vi "Material-Line1-Aquisition.vi"(8 "error in (no error)":errorcluster, 11 "Material-RunTest in":refnum<class "Material-RunTest.lvclass">) -> (0 "error out":errorcluster, 3 "Material-RunTest out":refnum<class "Material-RunTest.lvclass">)   [LabVIEW 2014, in "Material-RunTest.lvclass"]
uses:
  Material-RunTest.lvclass
  Material-RunTest.lvclass/Material-RunTest.ctl
  <instrlib>/Keyence LK-G5000/Public/enum/LKIF_OUTNO.ctl
  <vilib>/Utility/file.llb/Write To Spreadsheet File (DBL).vi
  <instrlib>/Keyence LK-G5000/Keyence LK-G5000.lvlib
  Motion Control/Motion-ControlAll.lvclass
  <vilib>/addons/_LabVIEW Style Book/Utilities/Style Book Utilities.lvlib
panel:
  out "Laser Value":sgl format="%_6g"
  out "Init Meas1":dbl[](array[numeric])
  out "stop collecting":bool=TRUE
  out "Meas 1 Dyn Data":dbl[](graph)
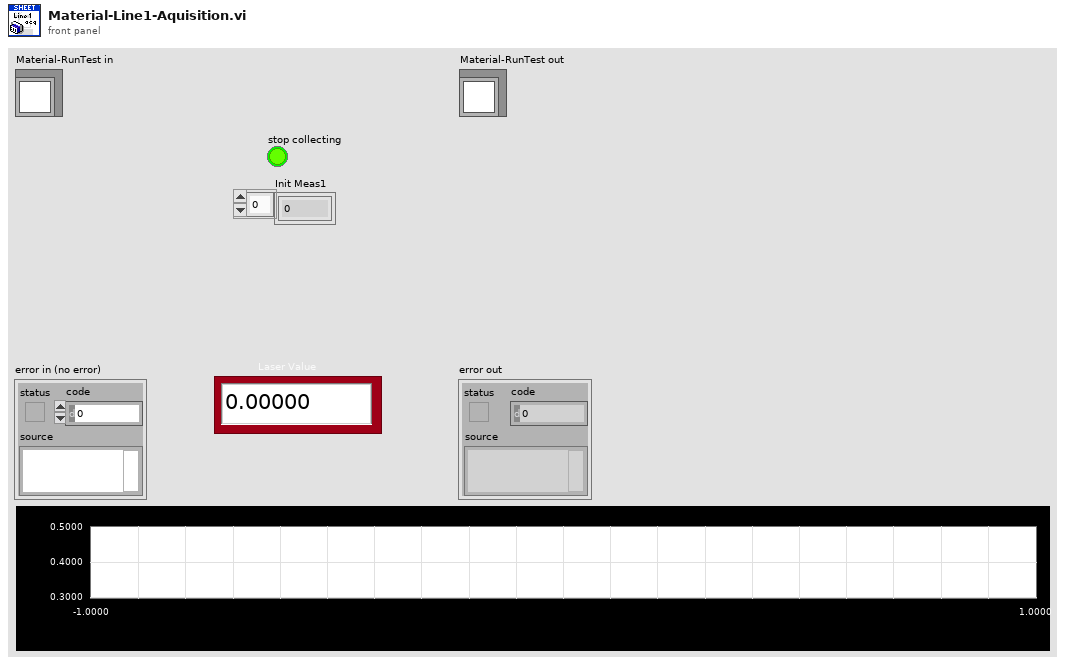
[diagram p1: front panel]
types:
  T1 = typedef "Keyence LK-G5000.lvlib/LKIF_OUTNO.ctl" = i32
  T2 = typedef "Keyence LK-G5000.lvlib/LKIF_FLOATRESULT.ctl" = i32
  T3 = cluster{"OutNo":i32, "LKIF_FLOATRESULT":T2, "Value":sgl}[]
  T4 = cluster{"OutNo":i32, "LKIF_FLOATRESULT":T2, "Value":sgl}
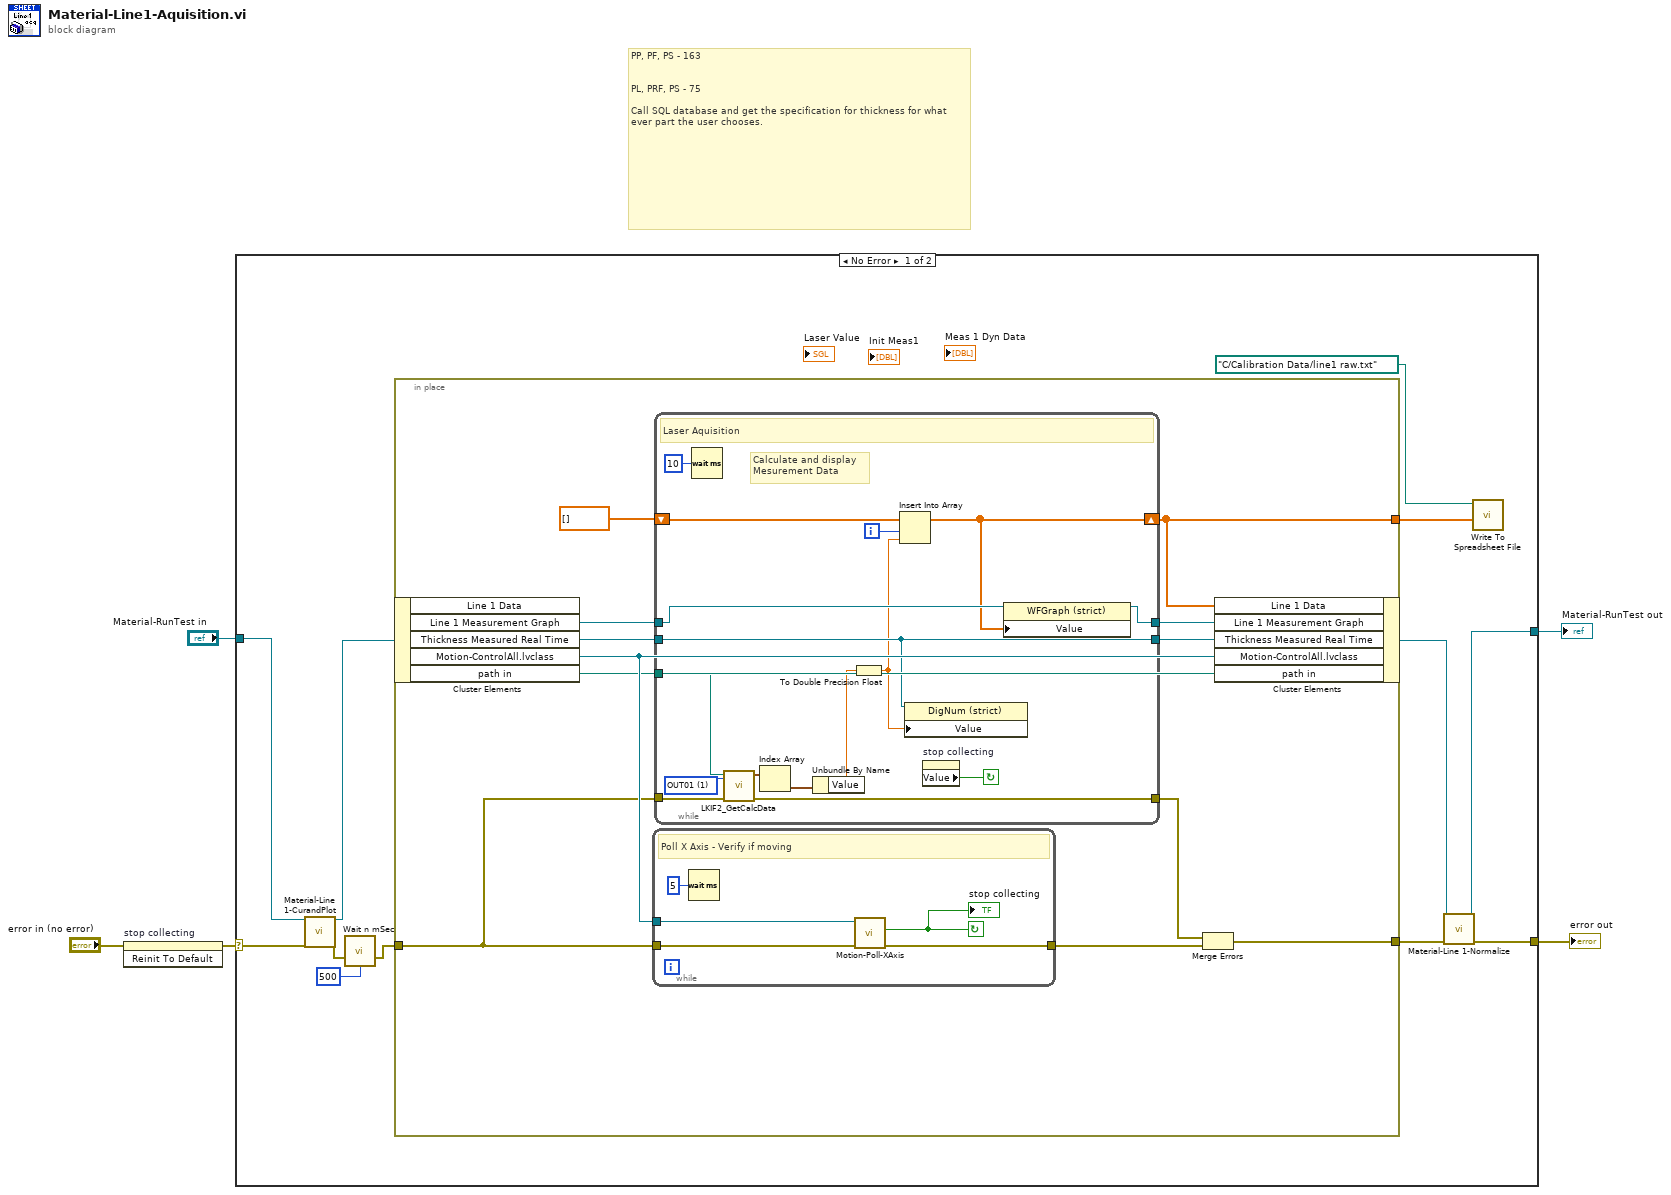
[diagram p0: block diagram]
diagram:
  # "PP, PF, PS - 163\n\n\nPL, PRF, PS - 75\n\nCall SQL database and get the specification for thickness for what ever part the user chooses."
  n1 = invoke on="stop collecting" class="Bool (strict)" method="Reinit To Default"(error in="error in (no error)") -> (error out=w1:errorcluster)  [unwired: 2 in, 2 out]
  n2 = case shown="No Error" w1 {
    selector: w1 -> [w16 w52]
    tunnel: [w11 w52] -> w5
    tunnel: [w12 w51] -> w3
    tunnel: "Material-RunTest in" -> [w17 w51]
    frame No Error {
      n3 = call "Material-Line 1-CurandPlot.vi"("Material-RunTest in"=w17, "error in (no error)"=w16) -> ("Material-RunTest out"=w15:refnum<class "Material-RunTest.lvclass">, "error out"=w9:errorcluster)  [unwired: 16 in]
      n4 = call <vilib>:"Wait n mSec.vi"("error in (no error)"=w9, "Milliseconds to Wait (500)"=u32 500) -> ("error out"=w8:errorcluster)  [unwired: 13 in]
      n5 = in-place {
        in-place-border: w8 -> [w19]
        in-place-border: [w23] -> w14
        in-place-border: [w18] -> w6
        n6 = in-place-cluster #1(w15) -> ("Line 1 Measurement Graph"=w21:refnum<vi>, "Thickness Measured Real Time"=w29:refnum<vi>, "Motion-ControlAll.lvclass"=w26:refnum<class "Motion-ControlAll.lvclass">, "path in"=w20:path)  [unwired: 1 out]
        n7 = while {
          tunnel: w19 -> [w33]
          tunnel: [w31] -> w25
          tunnel: w26 -> [w32]
          stop <- w30 continue-if-true
          # "Poll X Axis - Verify if moving"
          n8 = Wait (ms)(milliseconds to wait=u32 5) -> ()  [unwired: 1 out]
          n9 = call "Motion-Poll-XAxis.vi"("error in (no error)"=w33, "Motion-ControlAll in"=w32) -> ("error out"=w31:errorcluster, "X axis \nstopped"=w30:bool)  [unwired: 7 in, 1 out]
          "stop collecting" <- w30
        }
        n10 = while {
          tunnel: w19 -> [w50]
          tunnel: [w36] -> w24
          tunnel: w29 -> [w42]
          shift-right: [w37] -> w18
          shift-left: dbl[] [] -> [w45]
          tunnel: w21 -> [w44]
          tunnel: [w43] -> w28
          tunnel: [w42] -> w27
          tunnel: w20 -> [w35]
          i -> [w41]
          stop <- w40 continue-if-true
          w49 = T1 1 items=["OUT01"=1, "OUT02"=2, "OUT03"=4, "OUT04"=8, "OUT05"=16, "OUT06"=32, "OUT07"=64, "OUT08"=128, "OUT09"=256, "OUT10"=512, "OUT11"=1024, "OUT12"=2048, "ALL OUT"=4095] ("OutNo (OUT1)")
          # "Calculate and display \nMesurement Data"
          # "Laser Aquisition"
          n11 = Wait (ms)(milliseconds to wait=u32 10) -> ()  [unwired: 1 out]
          n12 = call <instrlib>:"LKIF2_GetCalcData.vi"("OutNo (OUT1)"=w49, "error in (no error)"=w50, "path in"=w35) -> ("error out"=w36:errorcluster, "CalcData"=w48:T3)  [unwired: 7 in]
          n13 = Index Array(array=w48) -> (element=w47:T4)  [unwired: 1 in]
          n14 = Unbundle By Name(w47) -> ("Value"=w39:sgl)
          n15 = To Double Precision Float(number=w39) -> (double precision float=w38:dbl)
          n16 = Insert Into Array(array=w45, index=w41, new element=w38) -> (w37:dbl[])
          n17 = property class="DigNum (strict)"(reference=w42, "Value"=w38) -> ()  [unwired: 1 in, 2 out]
          n18 = property on="stop collecting" class="Bool (strict)"() -> ("Value"=w40:bool)  [unwired: 2 in, 2 out]
          n19 = property class="WFGraph (strict)"(reference=w44, "Value"=w37) -> (reference out=w43:refnum<vi>)  [unwired: 1 in, 1 out]
        }
        n20 = Merge Errors(w24, w25) -> (w23:errorcluster)
        n21 = in-place-cluster #1("Line 1 Data"=w18, "Line 1 Measurement Graph"=w28, "Thickness Measured Real Time"=w27, "Motion-ControlAll.lvclass"=w26, "path in"=w20) -> (w13:refnum<class "Material-RunTest.lvclass">)
      }
      n22 = call "Material-Line 1-Normalize.vi"("error in (no error)"=w14, "Material-RunTest in"=w13) -> ("error out"=w11:errorcluster, "Material-RunTest out"=w12:refnum<class "Material-RunTest.lvclass">)  [unwired: 8 in]
      n23 = call-poly <vilib>:"Write To Spreadsheet File.vi"("1D data"=w6, "file path (dialog if empty)"=path "C:/Calibration Data/line1 raw.txt") -> ()  [unwired: 6 in, 1 out]
    }
    frame Error {
    }
  }
  "error out" <- w5
  "Material-RunTest out" <- w3
